vi "Process Data.vi"(8 "error in":errorcluster, 11 "Example GUI in":refnum<class "GUI.lvclass">) -> (0 "error out":errorcluster, 3 "Example GUI out":refnum<class "GUI.lvclass">)   [LabVIEW 2014, in "GUI.lvclass"]
uses:
  GUI.lvclass
  Architecture/Classes/Topic_class/Topic.lvclass
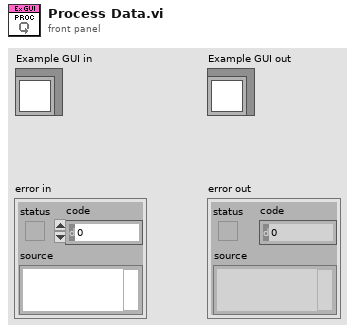
[diagram p1: front panel]
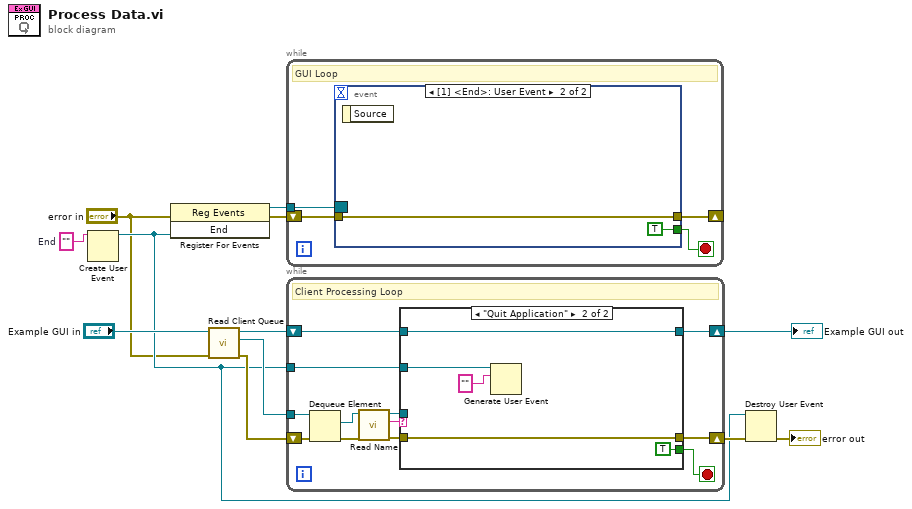
[diagram p0: block diagram]
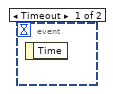
[diagram p3: hidden frame]
diagram:
  w11 = ""  # End
  n1 = Create User Event(user event datatype=w11) -> (user event=w5:refnum<user-event>)  [unwired: 1 in, 1 out]
  n2 = register-events(error in="error in", w5) -> (reference out=w10:refnum<event-registration>, error out=w1:errorcluster)  [unwired: 1 in]
  n3 = call-dynamic "Read Client Queue.vi"("error in"="error in", "Client in"="Example GUI in") -> ("error out"=w8:errorcluster, "Client Queue"=w9:refnum<queue>, "Client out"=w4:refnum<class "GUI.lvclass">)  [unwired: 7 in]
  n4 = while {
    tunnel: w10 -> [w16]
    shift-right: [w13] -> _
    shift-left: w1 -> [w14]
    stop <- w15 stop-if-true
    # "GUI Loop"
    n5 = event shown="[1] <End>: User Event" {
      selector: w16 -> [_ _]
      dyn-events: _ -> [_ _]
      timeout: _ -> [_ _]
      tunnel: [_ TRUE] -> w15
      tunnel: w14 -> [_ w17]
      tunnel: [_ w17] -> w13
      event Timeout {
        n6 = event-data() -> ()  [unwired: 1 in, 1 out]
      }
      event User Event {
        n7 = event-data() -> ()  [unwired: 1 in, 1 out]
      }
    }
  }
  n8 = while {
    tunnel: w9 -> [w28]
    shift-right: [w22] -> w7
    shift-left: w8 -> [w25]
    tunnel: w5 -> [w21]
    shift-right: [w19] -> w3
    shift-left: w4 -> [w20]
    stop <- w24 stop-if-true
    # "Client Processing Loop"
    n9 = Dequeue Element(queue=w28, error in (no error)=w25) -> (element=w29:refnum<class "Topic.lvclass">, error out=w30:errorcluster)  [unwired: 1 in, 2 out]
    n10 = call-dynamic "Read Name.vi"("error in"=w30, "Topic in"=w29) -> ("error out"=w23:errorcluster, "Name"=w27:string, "Topic out"=w26:refnum<class "Topic.lvclass">)  [unwired: 7 in]
    n11 = case shown="\"Quit Application\"" w27 {
      tunnel: w26 -> [_ _]
      tunnel: [_ TRUE] -> w24
      tunnel: w23 -> [w32 w36]
      tunnel: [w32 w36] -> w22
      tunnel: w21 -> [_ w34]
      tunnel: w20 -> [w31 w33]
      tunnel: [w31 w33] -> w19
      frame Default {
      }
      frame "Quit Application" {
        n12 = Generate User Event(user event=w34, event data cluster="" ("event data")) -> ()  [unwired: 2 in, 2 out]
      }
    }
  }
  "Example GUI out" <- w3
  n13 = Destroy User Event(user event=w5, error in=w7) -> (error out=→"error out":errorcluster)
